vi "Bool String.vi"(10 "Bool":bool) -> (2 "String":string)   [LabVIEW 2020, in "CTI-Visa.lvlib"]
uses:
  CTI-Visa.lvlib
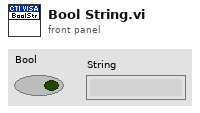
[diagram p1: front panel]
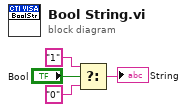
[diagram p0: block diagram]
diagram:
  n1 = Select(t="1", s="Bool", f="0") -> (s? t:f=→"String":string)
